vi "Utility Append to Build INI.vi"(8 "error in (no error)":errorcluster, 10 "Files Generated by Build":path[](array[path]), 11 "Project Path":path) -> (0 "error out":errorcluster)   [LabVIEW 2015]
doc: "Appends ini text to the end of the build INI file, copied from \"Post-Op Append.ini\""
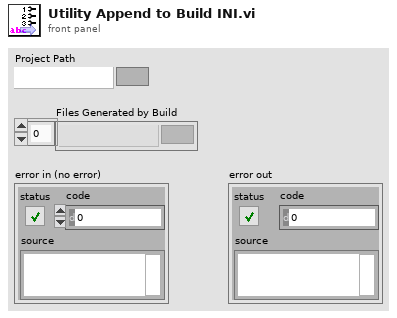
[diagram p1: front panel]
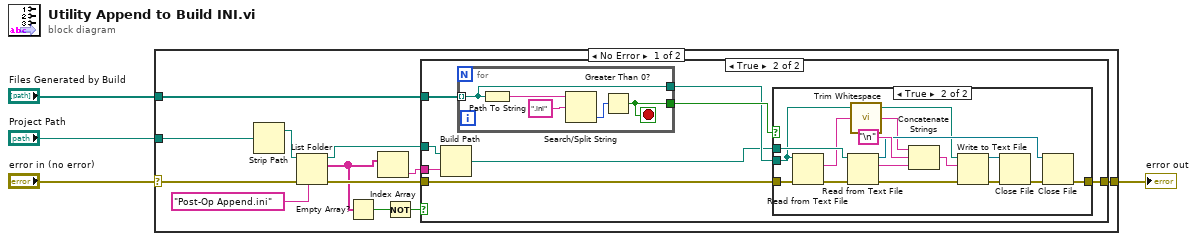
[diagram p0: block diagram]
diagram:
  n1 = case shown="No Error" "error in (no error)" {
    selector: "error in (no error)" -> [w11 w47]
    tunnel: [w12 w47] -> w4
    tunnel: "Project Path" -> [w10 _]
    tunnel: "Files Generated by Build" -> [w9 _]
    frame No Error {
      n2 = Strip Path(path=w10) -> (stripped path=w13:path)  [unwired: 1 out]
      n3 = List Folder(path=w13, pattern="Post-Op Append.ini", error in=w11) -> (path out=w15:path, filenames=w8:string[], error out=w16:errorcluster)  [unwired: 1 in, 1 out]
      n4 = Empty Array?(array=w8) -> (empty?=w7:bool)
      n5 = Index Array(array=w8) -> (element=w5:string)  [unwired: 1 in]
      n6 = Not(x=w7) -> (.not. x?=w6:bool)
      n7 = case shown="True" w6 {
        tunnel: w15 -> [_ w25]
        tunnel: [w17 w19] -> w12
        tunnel: w16 -> [w17 w18]
        tunnel: w9 -> [_ w23]
        tunnel: w5 -> [_ w24]
        frame False {
        }
        frame True {
          n8 = Build Path(base path=w25, name or relative path=w24) -> (appended path=w20:path)
          n9 = for {
            tunnel: w23 -> [w42] mode=indexing
            tunnel: [w43] -> w22
            tunnel: [w42] -> w21
            stop <- w43 stop-if-true
            n10 = Path To String(path=w42) -> (string=w46:string)
            n11 = Search/Split String(string=w46, search string/char (-)=".ini" ("regular expression")) -> (offset of match=w44:i32)  [unwired: 1 in, 2 out]
            n12 = Greater Than 0?(x=w44) -> (x > 0?=w43:bool)
          }
          n13 = case shown="True" w22 {
            tunnel: w21 -> [_ w28]
            tunnel: w20 -> [_ w41]
            tunnel: [w26 w29] -> w19
            tunnel: w18 -> [w26 w39]
            frame False {
            }
            frame True {
              n14 = Read from Text File(file (use dialog)=w28, error in=w39) -> (text=w36:string, error out=w40:errorcluster)  [unwired: 2 in, 2 out]
              n15 = Read from Text File(file (use dialog)=w41, error in=w40) -> (refnum out=w31:refnum<file>, text=w38:string, error out=w34:errorcluster)  [unwired: 2 in, 1 out]
              n16 = call <vilib>:"Trim Whitespace.vi"("string"=w36) -> ("trimmed string"=w27:string)  [unwired: 1 in]
              n17 = Concatenate Strings(w27, "\n", w38) -> (w35:string)
              n18 = Write to Text File(file (use dialog)=w28, text=w35, error in=w34) -> (refnum out=w33:refnum<file>, error out=w32:errorcluster)  [unwired: 1 in, 1 out]
              n19 = Close File(refnum=w33, error in=w32) -> (error out=w30:errorcluster)  [unwired: 1 out]
              n20 = Close File(refnum=w31, error in=w30) -> (error out=w29:errorcluster)  [unwired: 1 out]
            }
          }
        }
      }
    }
    frame Error {
    }
  }
  "error out" <- w4
